vi "myRIO_BRig_Host_formatData_getExp.vi"(11 "input_folderPath":string) -> (2 "output_ExpPrefix":string)   [LabVIEW 2014]
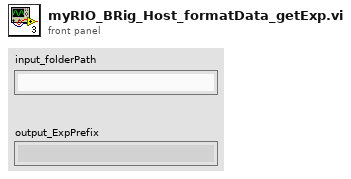
[diagram p1: front panel]
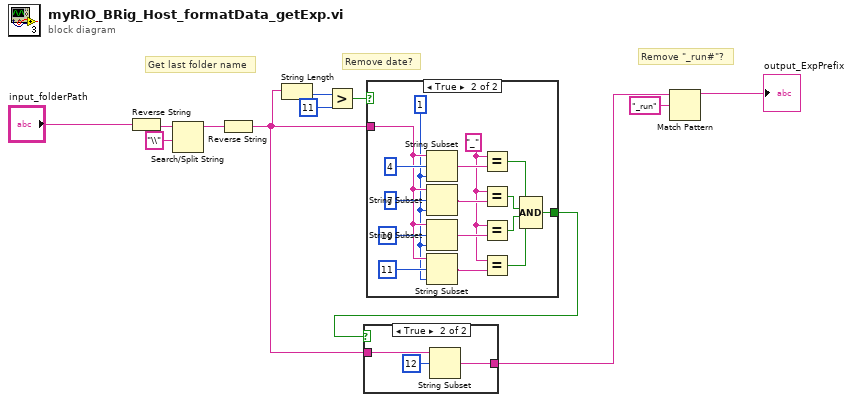
[diagram p0: block diagram]
diagram:
  # "Remove \"_run#\"?"
  # "Remove date?"
  # "Get last folder name"
  n1 = Reverse String(1:"input_folderPath") -> (0:w11:string)
  n2 = Search/Split String(string=w11, search string/char (-)="\\") -> (substring before match=w9:string)  [unwired: 1 in, 2 out]
  n3 = Reverse String(1:w9) -> (0:w4:string)
  n4 = String Length(string=w4) -> (length=w8:i32)
  n5 = Greater?(x=w8, y=11) -> (0:w6:bool)
  n6 = case shown="True" w6 {
    tunnel: w4 -> [_ w24]
    tunnel: [_ w14] -> w5
    frame False {
    }
    frame True {
      w13 = 1 ("length (rest)")
      w19 = "_" ("x")
      n7 = String Subset(string=w24, offset (0)=4, length (rest)=w13) -> (substring=w23:string)
      n8 = String Subset(string=w24, offset (0)=7, length (rest)=w13) -> (substring=w22:string)
      n9 = String Subset(string=w24, offset (0)=10, length (rest)=w13) -> (substring=w21:string)
      n10 = String Subset(string=w24, offset (0)=11, length (rest)=w13) -> (substring=w20:string)
      n11 = Equal?(x=w19, y=w23) -> (x = y?=w16:bool)
      n12 = Equal?(x=w19, y=w22) -> (x = y?=w18:bool)
      n13 = Equal?(x=w19, y=w21) -> (x = y?=w17:bool)
      n14 = Equal?(x=w19, y=w20) -> (x = y?=w15:bool)
      n15 = Compound Arithmetic op=AND(w16, w18, w17, w15) -> (w14:bool)
    }
  }
  n16 = case shown="True" w5 {
    tunnel: w4 -> [w29 w32]
    tunnel: [w29 w30] -> w3
    frame False {
    }
    frame True {
      n17 = String Subset(string=w32, offset (0)=12) -> (substring=w30:string)  [unwired: 1 in]
    }
  }
  n18 = Match Pattern(string=w3, regular expression="_run") -> (before substring=→"output_ExpPrefix":string)  [unwired: 1 in, 3 out]
